vi "Out_S5F3.vi"(8 "error in (no error)":errorcluster, 10 "S5F3":T1, 11 "S5 Message Class in":refnum<class "S5 Message Class.lvclass">) -> (0 "error out":errorcluster, 3 "S5 Message Class out":refnum<class "S5 Message Class.lvclass">)   [LabVIEW 2020, in "SECS Communication.lvlib" / "S5 Message Class.lvclass"]
uses:
  S5 Message Class.lvclass
  D:/Dropbox/SECS/LabVIEW Code/Com/SECS Communication/SECS-II Class/SECS-II Class.lvclass
  S5F3.ctl
  SECS-II Class/Data Message_List.vi
  SECS-II Class/Data Message_Binary.vi
  SECS-II Class/Data Message_U4.vi
  S5 Message Class.lvclass/S5 Message Class.ctl
  SECS-II Class/SECS-II Class.lvclass
  D:/Dropbox/SECS/LabVIEW Code/Com/SECS Communication/S5 Message Class/S5 Message Class.lvclass
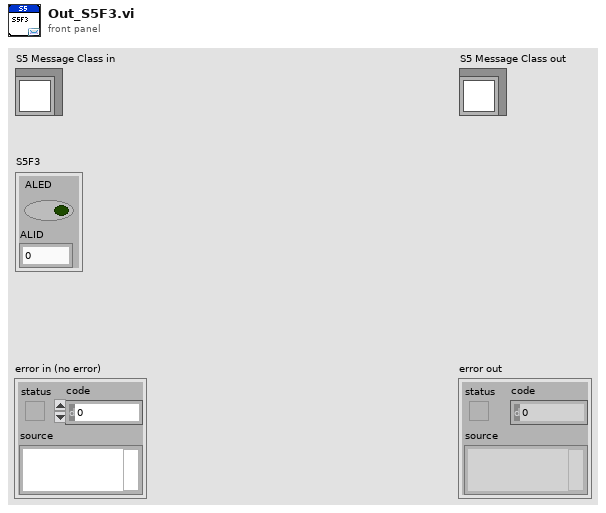
[diagram p1: front panel]
types:
  T1 = typedef "SECS Communication.lvlib/S5 Message Class.lvclass/S5F3.ctl" = cluster{"ALED":bool, "ALID":u32}
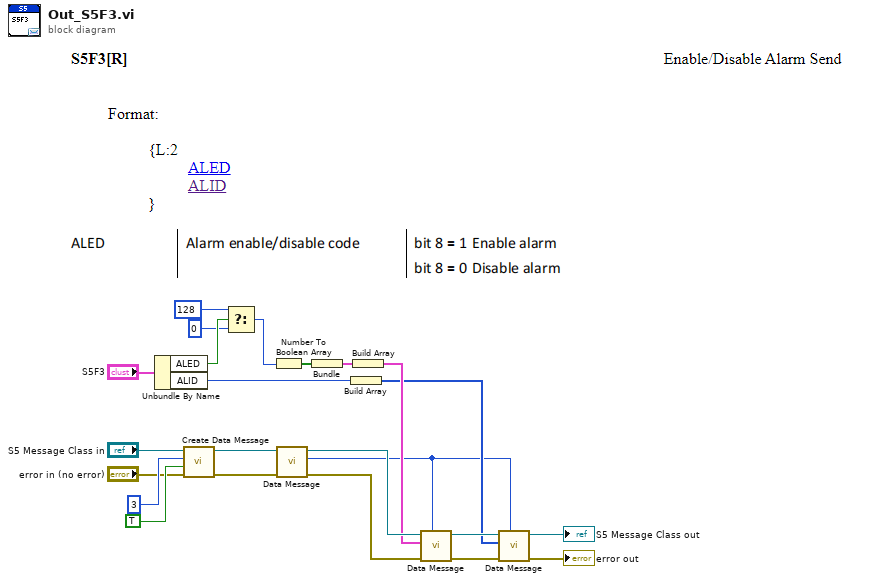
[diagram p0: block diagram]
diagram:
  n1 = Unbundle By Name("S5F3") -> ("ALED"=w4:bool, "ALID"=w9:u32)
  n2 = call "Create Data Message.vi"("error in (no error)"="error in (no error)", "W-Bit"=TRUE, "Function"=u8 3, "SECS-II Class in"="S5 Message Class in") -> ("error out"=w20:errorcluster, "SECS-II Class out"=w21:refnum<class "S5 Message Class.lvclass">)  [unwired: 6 in]
  n3 = Select(t=u8 128, s=w4, f=u8 0) -> (s? t:f=w1:u8)
  n4 = Number To Boolean Array(number=w1) -> (Boolean array=w14:bool[])
  n5 = call-poly "Data Message.vi"("error in"=w20, "SECS-II Class in"=w21) -> ("error out"=w17:errorcluster, "Index"=w7:i32, "SECS-II Class out"=w16:refnum<class "S5 Message Class.lvclass">)  [unwired: 7 in]
  n6 = Bundle("Boolean array"=w14) -> (w13:cluster{"Boolean array":bool[]})  [unwired: 1 in]
  n7 = Build Array(w9) -> (w8:u32[])
  n8 = Build Array(w13) -> (w12:cluster{"Boolean array":bool[]}[])
  n9 = call-poly "Data Message.vi"("Parent Index"=w7, "error in"=w17, "Data Cluster"=w12, "SECS-II Class in"=w16) -> ("error out"=w10:errorcluster, "SECS-II Class out"=w11:refnum<class "S5 Message Class.lvclass">)  [unwired: 6 in]
  n10 = call-poly "Data Message.vi"("Parent Index"=w7, "error in"=w10, "Data"=w8, "SECS-II Class in"=w11) -> ("error out"=→"error out":errorcluster, "SECS-II Class out"=→"S5 Message Class out":refnum<class "S5 Message Class.lvclass">)  [unwired: 6 in]
